vi "SlopeAndIntecept.vi"(11 "Array in":dbl[][](array[numeric])) -> (2 "Fit":dbl[](array[numeric]), 3 "Array out":cluster{dbl[], dbl[]}[](array[cluster]))   [LabVIEW 2020]
uses:
  <vilib>/Analysis/6fits.llb/Curve Fitting Criteria.ctl
  <vilib>/Utility/file.llb/Write Delimited Spreadsheet (DBL).vi
  <vilib>/Analysis/NI_AALPro.lvlib
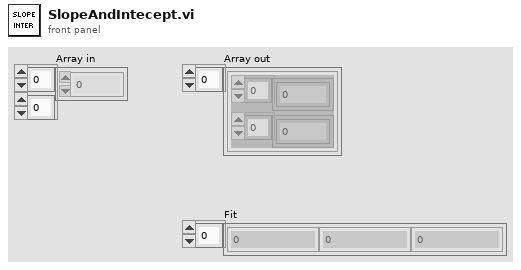
[diagram p1: front panel]
types:
  T1 = typedef "NI_AALPro.lvlib/Curve Fitting Criteria.ctl" = u16
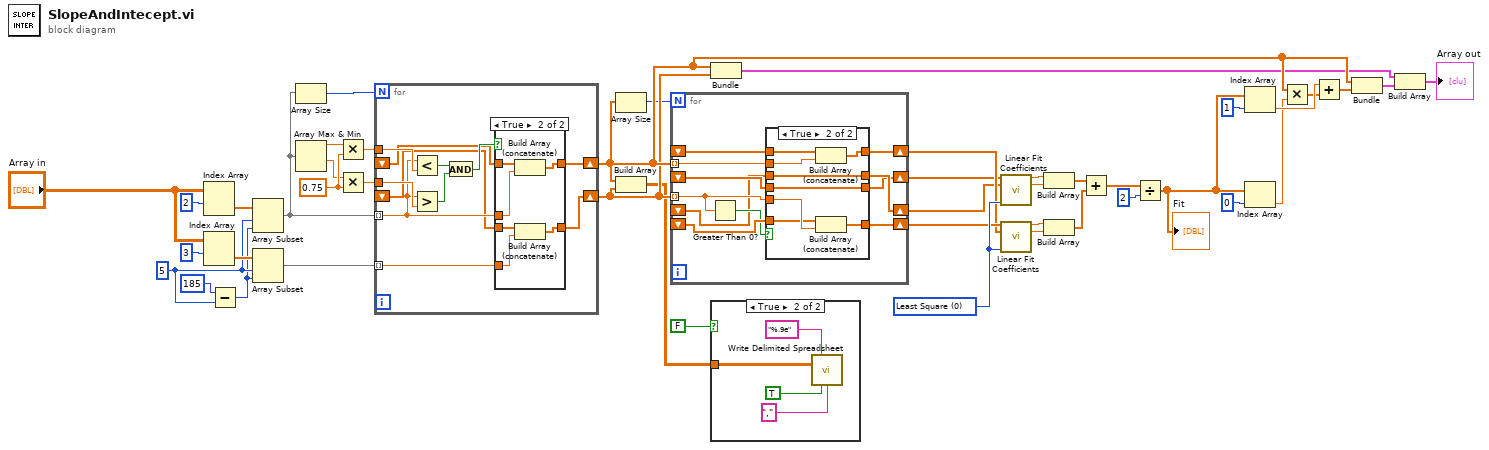
[diagram p0: block diagram]
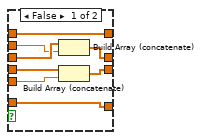
[diagram p2: hidden frame]
diagram:
  w19 = 0.75 ("y")
  w3 = 5 ("y")
  w33 = T1 0 items=["Least Square", "Least Absolute Residual", "Bisquare"] ("method")
  n1 = Index Array(array="Array in", index (row)=2) -> (element=w12:dbl[])  [unwired: 1 in]
  n2 = Index Array(array="Array in", index (row)=3) -> (element=w13:dbl[])  [unwired: 1 in]
  n3 = Subtract(x=185, y=w3) -> (x-y=w2:i32)
  n4 = Array Subset(array=w12, index=w3, length=w2) -> (w21:dbl[])
  n5 = Array Subset(array=w13, index=w3, length=w2) -> (w22:dbl[])
  n6 = Array Size(array=w21) -> (size(s)=w20:i32)
  n7 = Array Max & Min(array=w21) -> (max value=w17:dbl, min value=w18:dbl)  [unwired: 2 out]
  n8 = Multiply(x=w17, y=w19) -> (x*y=w23:dbl)
  n9 = Multiply(x=w18, y=w19) -> (x*y=w24:dbl)
  n10 = for {
    N: w20 -> [_]
    tunnel: w21 -> [w48] mode=indexing
    tunnel: w22 -> [w47] mode=indexing
    tunnel: w23 -> [w52]
    tunnel: w24 -> [w51]
    shift-right: [w49] -> w28
    shift-left: _ -> [w50]
    shift-right: [w46] -> w27
    shift-left: _ -> [w45]
    n11 = Less?(x=w48, y=w52) -> (x < y?=w55:bool)
    n12 = Greater?(x=w48, y=w51) -> (0:w53:bool)
    n13 = And(x=w55, y=w53) -> (x .and. y?=w54:bool)
    n14 = case shown="True" w54 {
      tunnel: w50 -> [w57 w62]
      tunnel: [w57 w63] -> w49
      tunnel: w48 -> [_ w61]
      tunnel: w47 -> [_ w60]
      tunnel: [w56 w59] -> w46
      tunnel: w45 -> [w56 w58]
      frame False {
      }
      frame True {
        n15 = Build Array (concatenate)(w62, w61) -> (w63:dbl[])
        n16 = Build Array (concatenate)(w58, w60) -> (w59:dbl[])
      }
    }
  }
  n17 = Array Size(array=w28) -> (size(s)=w26:i32)
  n18 = Build Array(w28, w27) -> (w16:dbl[][])
  n19 = for {
    N: w26 -> [_]
    tunnel: w28 -> [w72] mode=indexing
    tunnel: w27 -> [w69] mode=indexing
    shift-right: [w73] -> w31
    shift-left: _ -> [w74]
    shift-right: [w71] -> w32
    shift-left: _ -> [w70]
    shift-right: [w67] -> w29
    shift-left: _ -> [w64]
    shift-right: [w66] -> w30
    shift-left: _ -> [w65]
    n20 = Greater Than 0?(x=w69) -> (x > 0?=w68:bool)
    n21 = case shown="True" w68 {
      tunnel: w74 -> [w82 w89]
      tunnel: [w82 w90] -> w73
      tunnel: w72 -> [w76 w88]
      tunnel: w69 -> [w75 w87]
      tunnel: [w81 w86] -> w71
      tunnel: w70 -> [w81 w85]
      tunnel: [w80 w84] -> w67
      tunnel: [w79 w83] -> w66
      tunnel: w65 -> [w77 w83]
      tunnel: w64 -> [w78 w84]
      frame False {
        n22 = Build Array (concatenate)(w78, w76) -> (w80:dbl[])
        n23 = Build Array (concatenate)(w77, w75) -> (w79:dbl[])
      }
      frame True {
        n24 = Build Array (concatenate)(w89, w88) -> (w90:dbl[])
        n25 = Build Array (concatenate)(w85, w87) -> (w86:dbl[])
      }
    }
  }
  n26 = Bundle(w28, w27) -> (w9:cluster{dbl[], dbl[]})  [unwired: 1 in]
  n27 = case shown="True" FALSE {
    tunnel: w16 -> [_ w91]
    frame False {
    }
    frame True {
      n28 = call-poly <vilib>:"Write Delimited Spreadsheet.vi"("format (%.3f)"="%.9e", "2D data"=w91, "transpose? (no:F)"=TRUE, "delimiter (\\t)"="," ("delimiter (\\t)")) -> ()  [unwired: 10 in, 2 out]
    }
  }
  n29 = call <vilib>:"Linear Fit Coefficients.vi"("Y"=w30, "X"=w29, "method"=w33) -> ("slope"=w7:dbl, "intercept"=w6:dbl)  [unwired: 10 in, 1 out]
  n30 = call <vilib>:"Linear Fit Coefficients.vi"("Y"=w32, "X"=w31, "method"=w33) -> ("slope"=w34:dbl, "intercept"=w35:dbl)  [unwired: 10 in, 1 out]
  n31 = Build Array(w7, w6) -> (w14:dbl[])
  n32 = Build Array(w34, w35) -> (w37:dbl[])
  n33 = Add(x=w14, y=w37) -> (x+y=w36:dbl[])
  n34 = Divide(x=w36, y=2) -> (x/y=w39:dbl[])
  "Fit" <- w39
  n35 = Index Array(array=w39, index=1) -> (element=w43:dbl)
  n36 = Index Array(array=w39, index=0) -> (element=w42:dbl)
  n37 = Multiply(x=w28, y=w42) -> (x*y=w5:dbl[])
  n38 = Add(x=w43, y=w5) -> (x+y=w4:dbl[])
  n39 = Bundle(w28, w4) -> (w8:cluster{dbl[], dbl[]})  [unwired: 1 in]
  n40 = Build Array(w9, w8) -> (→"Array out":cluster{dbl[], dbl[]}[])
